vi "HEWH RLT Valve Bit Flip.vi"(8 "Error In":errorcluster, 10 "NewVal in":T1) -> (0 "Error Out":errorcluster, 3 "NewVal out":T1)   [LabVIEW 2019]
uses:
  Custom Instrument Control/MW100/Type Definitions/HEWH Solenoid Valve Status.ctl
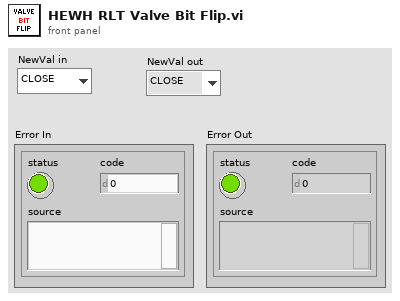
[diagram p1: front panel]
types:
  T1 = typedef "HEWH Solenoid Valve Status.ctl" = enum8{"CLOSE", "OPEN"}
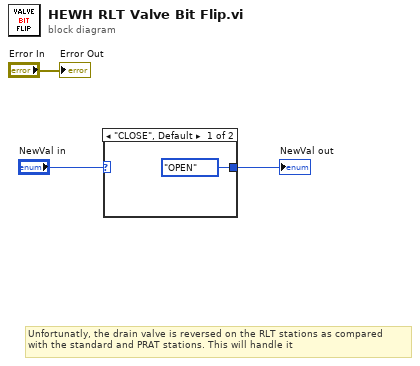
[diagram p0: block diagram]
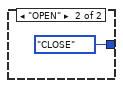
[diagram p2: hidden frame]
diagram:
  # "Unfortunatly, the drain valve is reversed on the RLT stations as compared\nwith the standard and PRAT stations. This will handle it"
  n1 = case shown="\"CLOSE\", Default" "NewVal in" {
    tunnel: [HEWH_Solenoid_Valve_Status."OPEN" ("NewVal") HEWH_Solenoid_Valve_Status."CLOSE" ("NewVal")] -> w3
    frame "CLOSE", Default {
    }
    frame "OPEN" {
    }
  }
  "NewVal out" <- w3
  "Error Out" <- "Error In"
